vi "ConPanes.vi"(8 "error in (no error)":errorcluster) -> (0 "error out":errorcluster)   [LabVIEW 2021, in "Markdown.lvlib"]
doc: "Exports the VI connector pane images."
uses:
  Markdown.lvlib
  Global.vi
  <vilib>/Utility/error.llb/Error Cluster From Error Code.vi
  <vilib>/ErrorRing/Error Ring.xnode
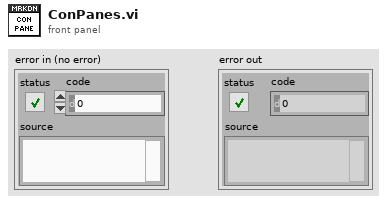
[diagram p1: front panel]
types:
  T1 = typedef "Markdown.lvlib/Item.ctl" = cluster{"Name":string, "Icon":picture, "Path":path, "Title":string, "Desc":string, "ConPane":picture, "TypeString":string, "ProjectItem":string, "VI Type":enum32{"invalid VI type", "Standard VI", "Control VI", "Global VI", "Polymorphic VI", "Configuration VI", "SubSystem", "Facade VI", "Method VI", "Statechart Diagram VI"}}
  T2 = enum32{"invalid VI type", "Standard VI", "Control VI", "Global VI", "Polymorphic VI", "Configuration VI", "SubSystem", "Facade VI", "Method VI", "Statechart Diagram VI"}
  T3 = typedef "imagedata.ctl" = cluster{"image type":i32, "image depth":i32, "image":u8[], "mask":u8[], "colors":u32[], "Rectangle":cluster{"left":i16, "top":i16, "right":i16, "bottom":i16}}
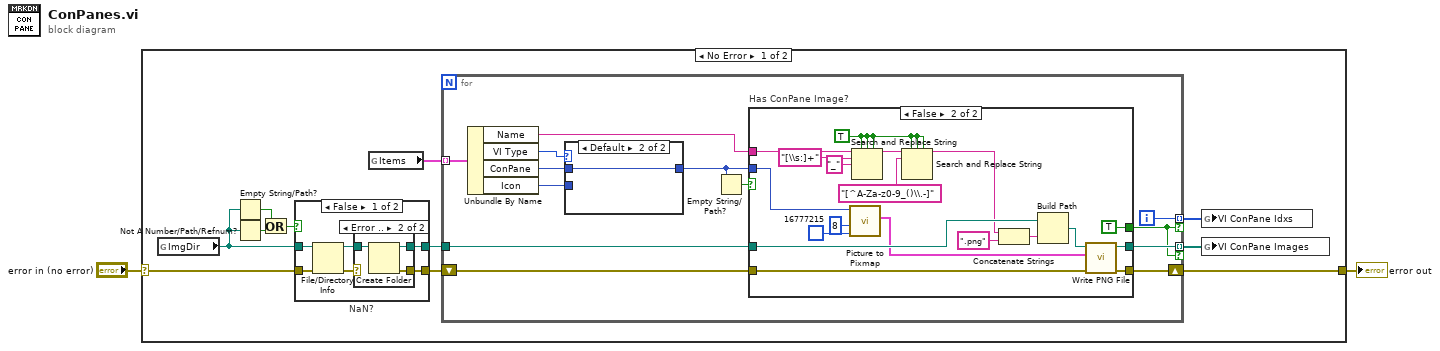
[diagram p0: block diagram]
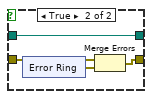
[diagram p3: hidden frame]
diagram:
  n1 = case shown="No Error" "error in (no error)" {
    selector: "error in (no error)" -> [w13 w68]
    tunnel: [w12 w68] -> w1
    frame No Error {
      n2 = global read "Global.vi" "ImgDir"() -> (w6:path)
      n3 = Empty String/Path?(string/path=w6) -> (empty?=w8:bool)
      n4 = Not A Number/Path/Refnum?(number/path/refnum=w6) -> (NaN/Path/Refnum?=w9:bool)
      n5 = Or(x=w8, y=w9) -> (x .or. y?=w7:bool)
      n6 = case "NaN?" shown="False" w7 {
        tunnel: w13 -> [w19 w28]
        tunnel: w6 -> [w17 w27]
        tunnel: [w16 w26] -> w11
        tunnel: [w14 w27] -> w10
        frame False {
          n7 = File/Directory Info(path=w17, error in=w19) -> (path out=w15:path, error out=w18:errorcluster)  [unwired: 5 out]
          n8 = case shown="Error .." w18 {
            selector: w18 -> [w20 _]
            tunnel: [w20 w24] -> w16
            tunnel: w15 -> [w21 w23]
            tunnel: [w21 w22] -> w14
            frame No Error {
            }
            frame Error {
              n9 = Create Folder(path (use dialog)=w23) -> (created path=w22:path, error out=w24:errorcluster)  [unwired: 2 in, 1 out]
            }
          }
        }
        frame True {
          n10 = xnode "Error Ring"() -> ("error out"=w25:errorcluster)
          n11 = Merge Errors(w28, w25) -> (w26:errorcluster)
        }
      }
      n12 = global read "Global.vi" "Items"() -> (w5:T1[])
      n13 = for {
        shift-right: [w45] -> w12
        shift-left: w11 -> [w39]
        tunnel: [w44] -> w3 mode=indexing if=w37
        tunnel: w10 -> [w43]
        tunnel: w5 -> [w42] mode=indexing
        tunnel: [w38] -> w4 mode=indexing if=w37
        i -> [w38]
        n14 = Unbundle By Name(w42) -> ("Name"=w40:string, "VI Type"=w34:T2, "ConPane"=w35:picture, "Icon"=w33:picture)
        n15 = case shown="Default" w34 {
          tunnel: [w46 w47] -> w36
          tunnel: w35 -> [_ w47]
          tunnel: w33 -> [w46 _]
          frame "Control VI".."Polymorphic VI" {
          }
          frame Default {
          }
        }
        n16 = Empty String/Path?(string/path=w36) -> (empty?=w41:bool)
        n17 = case "Has ConPane Image?" shown="False" w41 {
          tunnel: w39 -> [w48 w63]
          tunnel: [w48 w67] -> w45
          tunnel: [_ w65] -> w44
          tunnel: w43 -> [_ w64]
          tunnel: w40 -> [_ w50]
          tunnel: w36 -> [_ w52]
          tunnel: [_ TRUE] -> w37
          frame True {
          }
          frame False {
            w53 = TRUE ("replace all? (F)")
            n18 = call <vilib>:"Picture to Pixmap.vi"("Background Color"=u32 16777215, "depth"=8, "picture"=w52) -> ("image data"=w51:T3)  [unwired: 7 in, 1 out]
            n19 = Search and Replace String(replace all?=w53, case sensitive?=w53, multiline?=w53, input string=w50, search string="[\\s:]+", replace string="_" ("replace string (\"\")")) -> (result string=w56:string)  [unwired: 2 in, 3 out]
            n20 = Search and Replace String(replace all?=w53, case sensitive?=w53, multiline?=w53, input string=w56, search string="[^A-Za-z0-9_()\\.-]") -> (result string=w57:string)  [unwired: 3 in, 3 out]
            n21 = Concatenate Strings(w57, ".png" ("string")) -> (w49:string)
            n22 = Build Path(base path=w64, name or relative path=w49) -> (appended path=w66:path)
            n23 = call <vilib>:"Write PNG File.vi"("error in (no error)"=w63, "image data"=w51, "path to PNG file"=w66) -> ("error out"=w67:errorcluster, "path"=w65:path)  [unwired: 7 in]
          }
        }
      }
      n24 = global write "Global.vi" "VI ConPane Idxs"(w4) -> ()
      n25 = global write "Global.vi" "VI ConPane Images"(w3) -> ()
    }
    frame Error {
    }
  }
  "error out" <- w1
